vi "Common_Extra_Chs.vi"() -> (0 "Common Extra Channels":string[](array[string]))   [LabVIEW 2018]
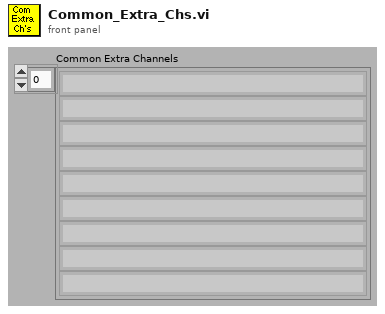
[diagram p1: front panel]
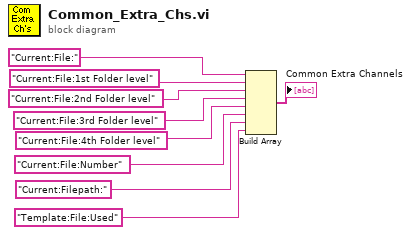
[diagram p0: block diagram]
diagram:
  n1 = Build Array("Current:File:", "Current:File:1st Folder level", "Current:File:2nd Folder level", "Current:File:3rd Folder level", "Current:File:4th Folder level", "Current:File:Number", "Current:Filepath:", "Template:File:Used") -> (→"Common Extra Channels":string[])
